vi "moveNodeUpDown.vi"(8 "error in (no error)":errorcluster, 9 "Direction":T1, 10 "subNode* in":refnum<data-value>, 11 "superNode in":refnum<class "xceNode.lvclass">) -> (0 "error out":errorcluster, 1 "No Change":bool, 2 "new Index":i32, 3 "superNode out":refnum<class "xceNode.lvclass">)   [LabVIEW 2013, in "xceNode.lvclass"]
doc: "Moves a nodes postion up in the subNode array of its superNode. Used to rearrange nodes with the same superNode."
uses:
  xceNode.lvclass
  xceTreeObj/xceTreeObj.lvclass
  xceRootNode/moveDirection.ctl
  xceNode.lvclass/xceNode.ctl
  xceRootNode/xceRootNode.lvclass
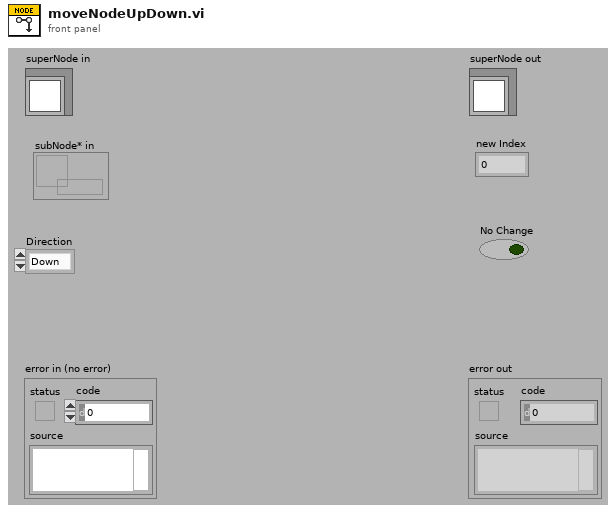
[diagram p1: front panel]
types:
  T1 = typedef "xceRootNode.lvclass/moveDirection.ctl" = enum16{"Down", "Up"}
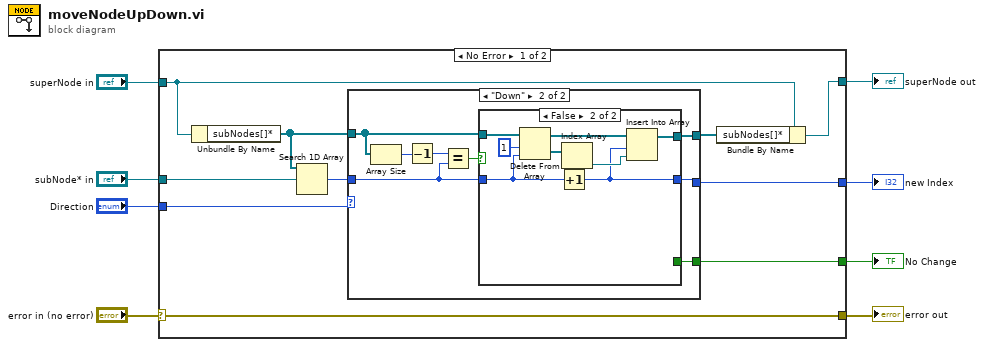
[diagram p0: block diagram]
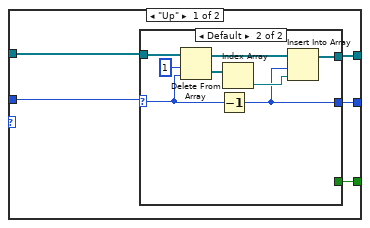
[diagram p2: hidden frame]
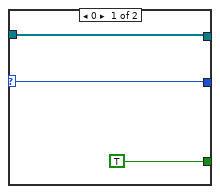
[diagram p3: hidden frame]
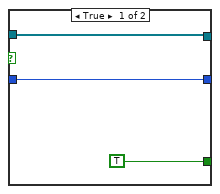
[diagram p4: hidden frame]
diagram:
  n1 = case shown="No Error" "error in (no error)" {
    selector: "error in (no error)" -> [w18 w55]
    tunnel: [w18 w55] -> w7
    tunnel: [w11 w54] -> w5
    tunnel: "superNode in" -> [w12 w54]
    tunnel: "Direction" -> [w16 _]
    tunnel: "subNode* in" -> [w17 _]
    tunnel: [w14 _] -> w2
    tunnel: [w9 _] -> w1
    frame No Error {
      n2 = Unbundle By Name(w12) -> ("subNodes[]*"=w10:refnum<data-value>[])
      n3 = Search 1D Array(1D array=w10, element=w17) -> (index of element=w15:i32)  [unwired: 1 in]
      n4 = case shown="\"Down\"" w16 {
        tunnel: w10 -> [w21 w40]
        tunnel: w15 -> [w23 w37]
        tunnel: [w22 w42] -> w14
        tunnel: [w20 w41] -> w13
        tunnel: [w19 w35] -> w9
        frame "Up" {
          n5 = case shown="Default" w23 {
            selector: w23 -> [w24 w29]
            tunnel: [TRUE _] -> w22
            tunnel: w21 -> [w25 w34]
            tunnel: [w25 w28] -> w20
            tunnel: [w24 w27] -> w19
            frame 0 {
            }
            frame Default {
              n6 = Delete From Array(array=w34, length=1, index=w29) -> (deleted portion=w32:refnum<data-value>[], array with subset deleted=w31:refnum<data-value>[])
              n7 = Decrement(x=w29) -> (x-1=w27:i32)
              n8 = Index Array(array=w32) -> (element=w30:refnum<data-value>)  [unwired: 1 in]
              n9 = Insert Into Array(array=w31, index=w27, new element=w30) -> (w28:refnum<data-value>[])
            }
          }
        }
        frame "Down" {
          n10 = Array Size(array=w40) -> (size(s)=w39:i32)
          n11 = Decrement(x=w39) -> (x-1=w38:i32)
          n12 = Equal?(x=w38, y=w37) -> (x = y?=w36:bool)
          n13 = case shown="False" w36 {
            tunnel: [TRUE _] -> w42
            tunnel: w40 -> [w44 w53]
            tunnel: [w44 w48] -> w41
            tunnel: w37 -> [w43 w47]
            tunnel: [w43 w46] -> w35
            frame True {
            }
            frame False {
              n14 = Delete From Array(array=w53, length=1, index=w47) -> (deleted portion=w51:refnum<data-value>[], array with subset deleted=w50:refnum<data-value>[])
              n15 = Increment(x=w47) -> (x+1=w46:i32)
              n16 = Index Array(array=w51) -> (element=w49:refnum<data-value>)  [unwired: 1 in]
              n17 = Insert Into Array(array=w50, index=w46, new element=w49) -> (w48:refnum<data-value>[])
            }
          }
        }
      }
      n18 = Bundle By Name(cluster=w12, "subNodes[]*"=w13) -> (w11:refnum<class "xceNode.lvclass">)
    }
    frame Error {
    }
  }
  "error out" <- w7
  "superNode out" <- w5
  "No Change" <- w2
  "new Index" <- w1
